vi "Limit Configuration.vi"(8 "error in (no error)":errorcluster caption="错误输入（无错误）", 11 "Limit Configuration":T1) -> (0 "error out":errorcluster caption="错误输出", 3 "Limit Configuration 2":T1)   [LabVIEW 2015, in "Boimetry Processing.lvlib"]
doc: "读取判断生物参数结果标准的设置值。"
uses:
  Boimetry Processing.lvlib
  Controls/Limit Configuration.ctl
  Utility VIs/Utility VIs.lvlib
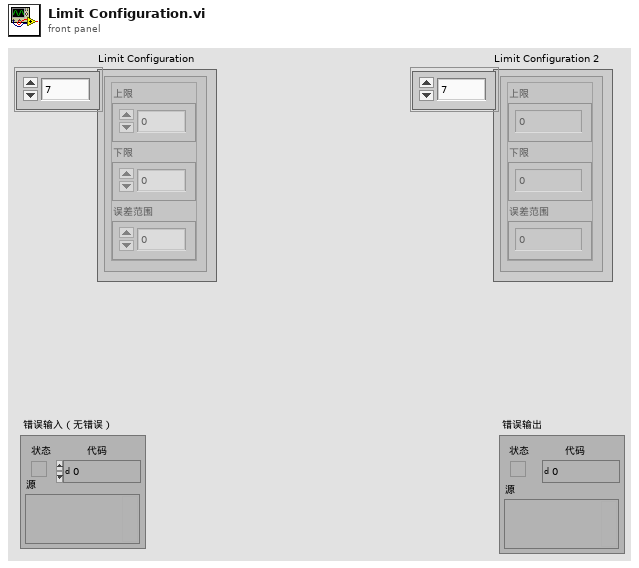
[diagram p1: front panel]
types:
  T1 = typedef "Boimetry Processing.lvlib/Limit Configuration.ctl" = cluster{"上限":dbl, "下限":dbl, "误差范围":dbl}[]
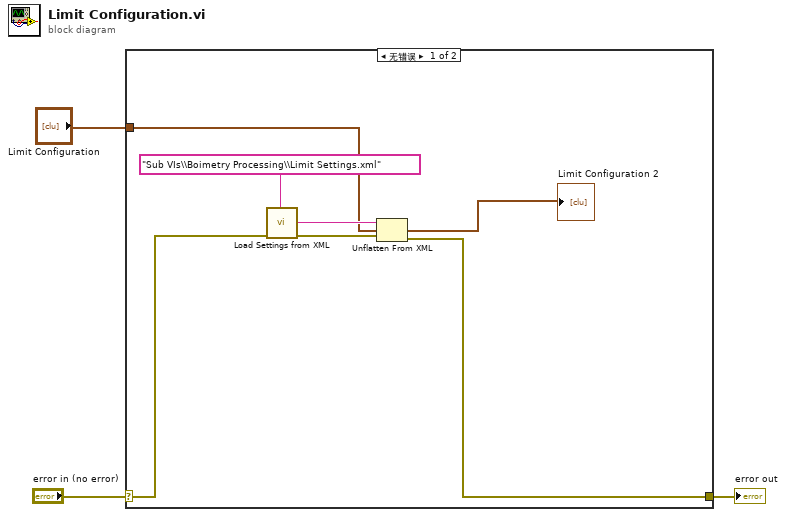
[diagram p0: block diagram]
diagram:
  n1 = case shown="无错误" "error in (no error)" {
    selector: "error in (no error)" -> [w6 w11]
    tunnel: [w5 w11] -> w2
    tunnel: "Limit Configuration" -> [w8 _]
    frame No Error {
      n2 = call "Load Settings from XML.vi"("error in (no error)"=w6, "名称或相对路径"="Sub VIs\\Boimetry Processing\\Limit Settings.xml") -> ("error out"=w7:errorcluster, "XML Elements"=w9:string)  [unwired: 8 in]
      n3 = Unflatten From XML(xml string=w9, type=w8, error in (no error)=w7) -> (value=→"Limit Configuration 2":T1, error out=w5:errorcluster)
    }
    frame Error {
    }
  }
  "error out" <- w2
